vi "Feasa Read Blinking, Colour, Intensity with Options.vi"(0 "VISA in":refnum<visa-resource-name>="COM12", 1 "Capture Time (ms)":i32=200 min=1 max=999, 2 "Exposure Factor":i32=1 caption="(00-15)" format="%02.0f", 3 "Wait Time between Capture (ms)":i32 min=0 max=999, 4 "Number of Capture":i32=20 min=0 max=9999, 5 "error in (no error)":errorcluster, 6 "Fiber Num":T1(ring)=enum."1", 7 "Lower Limit":dbl=2000.0 format="%#_13g", 8 "Maximum/Average/Minimum":enum16{"Maximum", "Average", "Minimum"}(ring), 9 "Upper Limit":dbl=5000.0 format="%#_13g") -> (10 "RED?":bool, 11 "Intensity":i32, 12 "GREEN?":bool, 14 "YELLOW?":bool, 15 "Blinking?":bool, 17 "ON?":bool, 18 "OFF?":bool, 19 "error out":errorcluster)   [LabVIEW 2025]
doc: "This VI is to for LED testwith using FEASA sequence mode.\n\nInput:\n- VISA in:\n Comm port in.\n\n- Fiber Num:\n Select Fiber Number to test. Fiber 1 to 10 channel. (can use for LED Analyser in 3F and 10F) \n\n- Capture Time (ms):\n Set capture time in milliseconds. \n (Note : This depends on the brightness of the LED. If the LED is dim then 1mS will cause the Analyser to be under-range. This could be determined by experiment.)\n\n- Wait Time between capture (ms):\n Set Wait time between Capture in milliseconds. \n\n- Number of Capture:\n Set a number of capture.\n\n- Maximum/Average/Minimum:\n Select intensity data and Wavelength to show in maximum value, average or minimum value. Default is maximum value.\n\n- Error in:\n Error message in.\n\nOutput:\n- Wavelength:\n Wavelength measurement (nm).\n\n- Intensity:\n Intensity measurement in count. This is relative intensity.\n\n- Status:\n Sending command process status.\n True : Passed\n False : Failed\n\n- LED Color:\n 1) RED?\n True: Yes.\n False: No.\n 2) GREEN?\n True: Yes.\n False: No.\n 3) BLUE?\n True: Yes.\n False: No.\n\n- LED Status:\n 1) Blinking?\n True: Yes.\n False: No.\n 2) ON?\n True: Yes.\n False: No.\n 3) OFF?\n True: Yes.\n False: No.\n\n- Error out:\n Error message out."
panel:
  out "Wavelength":i32
  out "Intensity (Min)":i32
  out "Wavelength (Min)":i32
  out "Wavelength (Ave)":dbl
  out "Wavelength (Max)":i32
  out "Intensity (Ave)":dbl
  out "Intensity (Max)":i32
  out "Status":bool
  out "Wavelength & Intensity":string
  # "LED Color"
  # "LED Status"
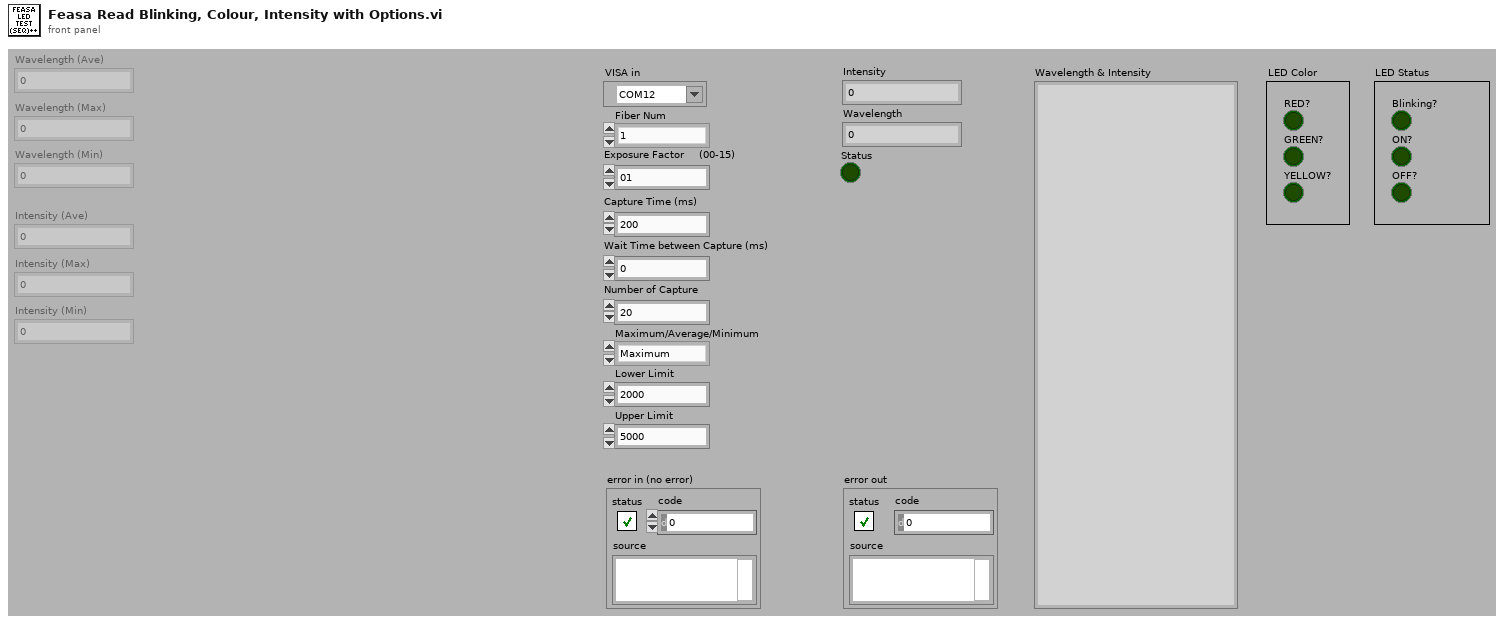
[diagram p1: front panel]
types:
  T1 = enum16{"All", "1", "2", "3", "4", "5", "6", "7", "8", "9", "10"}
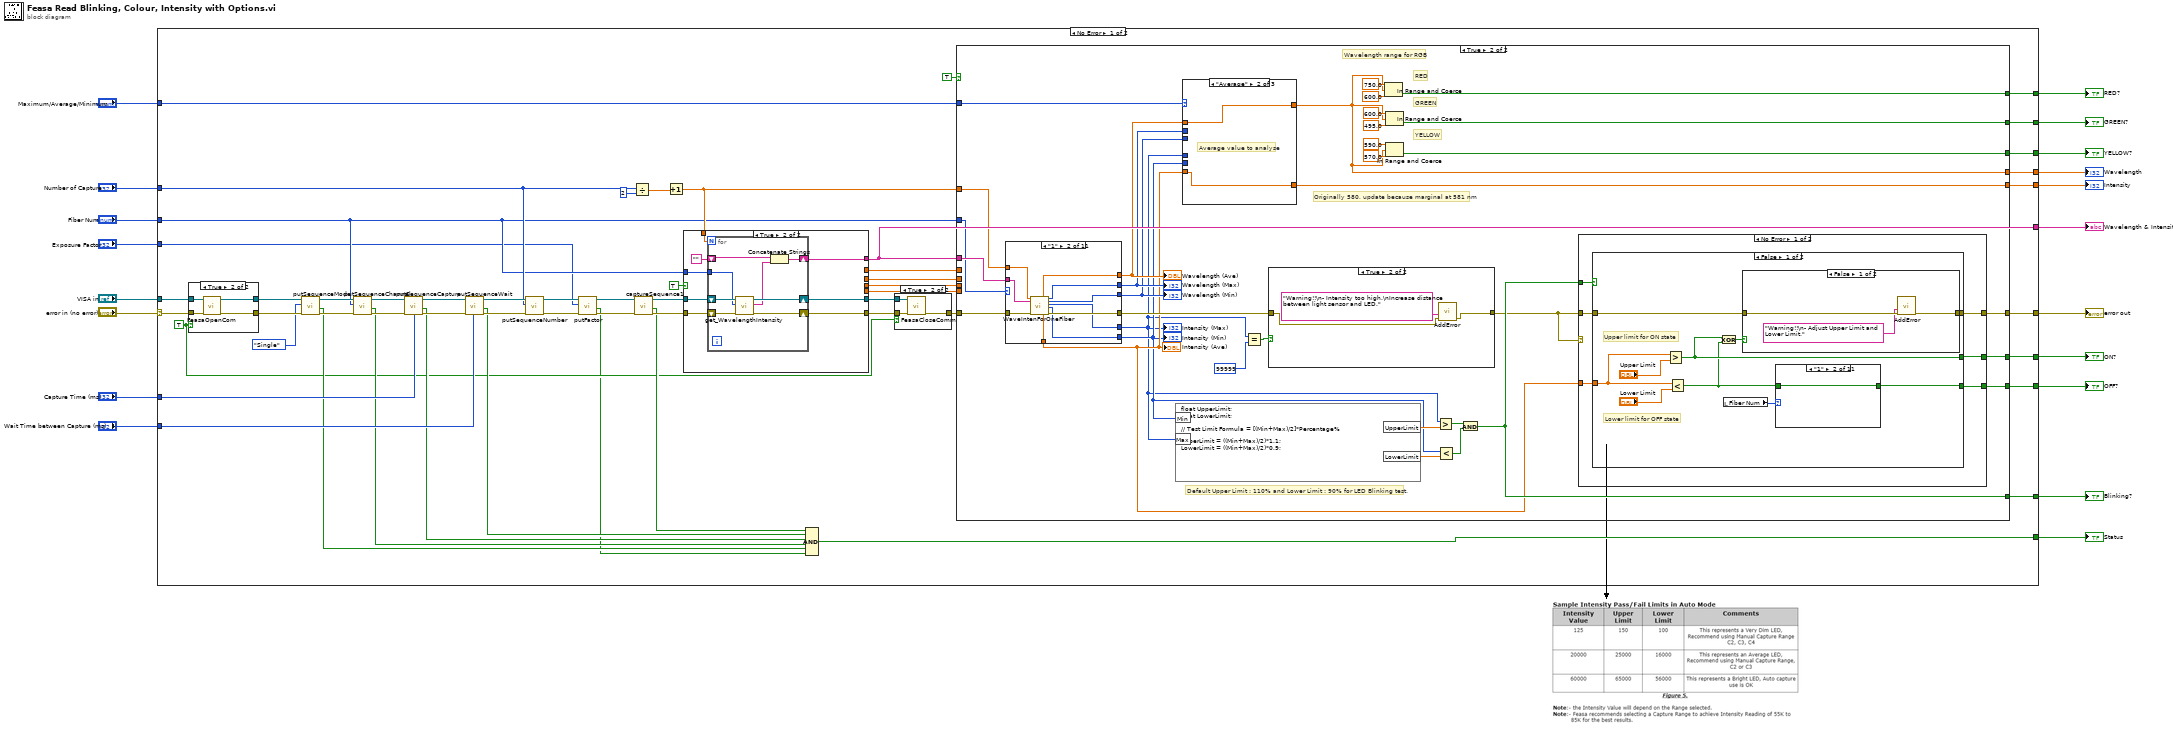
[diagram p0: block diagram]
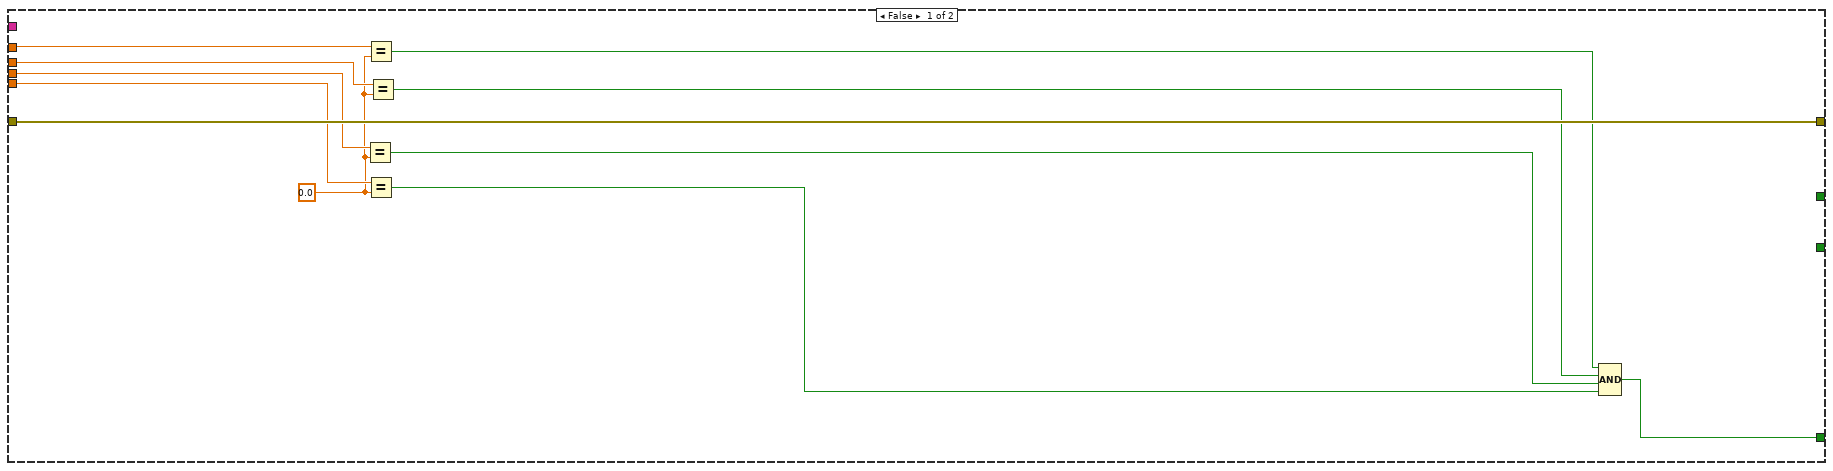
[diagram p4: hidden frame]
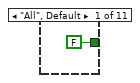
[diagram p5: hidden frame]
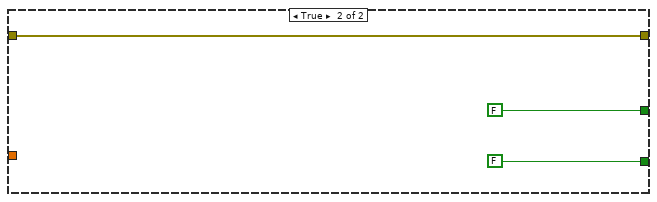
[diagram p16: hidden frame]
diagram:
  n1 = case shown="No Error" "error in (no error)" {
    selector: "error in (no error)" -> [w73 w301]
    tunnel: "VISA in" -> [w74 _]
    tunnel: [w41 w301] -> w17
    tunnel: "Fiber Num" -> [w36 _]
    tunnel: "Capture Time (ms)" -> [w70 _]
    tunnel: "Wait Time between Capture (ms)" -> [w67 _]
    tunnel: "Number of Capture" -> [w60 _]
    tunnel: [w52 _] -> w12
    tunnel: [w54 _] -> w11
    tunnel: "Maximum/Average/Minimum" -> [w50 _]
    tunnel: [w49 _] -> w9
    tunnel: [w48 _] -> w8
    tunnel: [w47 _] -> w7
    tunnel: [w46 _] -> w6
    tunnel: [w45 _] -> w5
    tunnel: [w44 _] -> w4
    tunnel: [w43 _] -> w3
    tunnel: [w42 _] -> w2
    tunnel: "Exposure Factor" -> [w21 _]
    frame No Error {
      w26 = TRUE
      n2 = case shown="True" w26 {
        tunnel: w74 -> [w79 w84]
        tunnel: w73 -> [w80 w83]
        tunnel: [w79 w82] -> w72
        tunnel: [w80 w81] -> w71
        frame False {
        }
        frame True {
          n3 = call "FeasaOpenCom.vi"("error in (no error)"=w83, "VISA resource name"=w84) -> ("error out"=w81:errorcluster, "VISA out"=w82:refnum<visa-resource-name>)  [unwired: 8 in]
        }
      }
      n4 = call "putSequenceMode.vi"("error in"=w71, "Sequence Mode"=enum16{"All", "Single"}."Single", "VISA in"=w72) -> ("error out"=w39:errorcluster, "Status"=w34:bool, "VISA out"=w37:refnum<visa-resource-name>)  [unwired: 6 in]
      n5 = call "putSequenceChannel.vi"("error in"=w39, "Fiber Num"=w36, "VISA in"=w37) -> ("error out"=w38:errorcluster, "Status"=w33:bool, "VISA out"=w35:refnum<visa-resource-name>)  [unwired: 6 in]
      n6 = call "putSequenceCapture.vi"("error in"=w38, "Millisecond (ms)"=w70, "VISA in"=w35) -> ("error out"=w68:errorcluster, "Status"=w55:bool, "VISA out"=w69:refnum<visa-resource-name>)  [unwired: 6 in]
      n7 = call "putSequenceWait.vi"("error in"=w68, "Millisecond (ms)"=w67, "VISA in"=w69) -> ("error out"=w65:errorcluster, "Status"=w56:bool, "VISA out"=w66:refnum<visa-resource-name>)  [unwired: 6 in]
      n8 = call "putSequenceNumber.vi"("error in"=w65, "Number to Capture"=w60, "VISA in"=w66) -> ("error out"=w22:errorcluster, "VISA out"=w25:refnum<visa-resource-name>)  [unwired: 6 in, 1 out]
      n9 = call "putFactor.vi"("error in"=w22, "Exposure Factor"=w21, "VISA in"=w25) -> ("error out"=w23:errorcluster, "Status"=w20:bool, "VISA out"=w24:refnum<visa-resource-name>)  [unwired: 6 in]
      n10 = Divide(x=w60, y=2) -> (x/y=w58:dbl)
      n11 = call "captureSequence1.vi"("error in"=w23, "VISA in"=w24) -> ("error out"=w62:errorcluster, "Status"=w57:bool, "VISA out"=w64:refnum<visa-resource-name>)  [unwired: 7 in]
      n12 = Increment(x=w58) -> (x+1=w51:dbl)
      n13 = case shown="True" TRUE {
        tunnel: w64 -> [w282 w292]
        tunnel: [w280 w291] -> w63
        tunnel: w62 -> [w283 w290]
        tunnel: [w284 w289] -> w61
        tunnel: [_ w287] -> w52
        tunnel: w51 -> [_ w286]
        tunnel: w36 -> [w281 w285]
        tunnel: [w279 _] -> w30
        tunnel: [w278 _] -> w29
        tunnel: [w277 _] -> w28
        tunnel: [w276 _] -> w27
        frame False {
          n14 = call "getflicker.vi"("VISA resource name"=w282, "fiber number"=w281, "error in"=w283) -> ("dup VISA resource name"=w280:refnum<visa-resource-name>, "Flicker %"=w279:dbl, "Flicker index"=w278:dbl, "Flicker Frequencies 1"=w277:dbl, "Flicker Frequencies 2"=w276:dbl, "error out"=w284:errorcluster)  [unwired: 11 in]
        }
        frame True {
          n15 = for {
            N: w286 -> [_]
            shift-right: [w299] -> w291
            shift-left: w292 -> [w300]
            shift-right: [w297] -> w289
            shift-left: w290 -> [w298]
            shift-right: [w294] -> w287
            shift-left: "" -> [w296]
            tunnel: w285 -> [w293]
            n16 = call "get_WavelengthIntensity.vi"("error in"=w298, "Fiber Num"=w293, "VISA in"=w300) -> ("error out"=w297:errorcluster, "WAVELENGTH INTENSITY"=w295:string, "VISA out"=w299:refnum<visa-resource-name>)  [unwired: 6 in]
            n17 = Concatenate Strings(w296, w295) -> (w294:string)
          }
        }
      }
      n18 = Compound Arithmetic op=AND(w57, w56, w55, w33, w34, w20) -> (w54:bool)
      n19 = case shown="True" w26 {
        tunnel: w63 -> [_ w78]
        tunnel: w61 -> [w75 w77]
        tunnel: [w75 w76] -> w53
        frame False {
        }
        frame True {
          n20 = call "FeasaCloseComm.vi"("error in"=w77, "VISA in:"=w78) -> ("error out"=w76:errorcluster)  [unwired: 9 in]
        }
      }
      n21 = case shown="True" TRUE {
        tunnel: w53 -> [w95 w129]
        tunnel: w52 -> [_ w128]
        tunnel: w51 -> [_ w127]
        tunnel: w50 -> [_ w121]
        tunnel: [_ w116] -> w49
        tunnel: [_ w115] -> w48
        tunnel: [_ w114] -> w47
        tunnel: [_ w113] -> w46
        tunnel: [_ w112] -> w45
        tunnel: [w89 w106] -> w44
        tunnel: [_ w104] -> w43
        tunnel: [_ w103] -> w42
        tunnel: [w95 w101] -> w41
        tunnel: w36 -> [_ w96]
        tunnel: w30 -> [w94 _]
        tunnel: w29 -> [w93 _]
        tunnel: w28 -> [w92 _]
        tunnel: w27 -> [w91 _]
        frame False {
          w90 = 0.0 ("y")
          n22 = Equal?(x=w92, y=w90) -> (x = y?=w86:bool)
          n23 = Equal?(x=w94, y=w90) -> (x = y?=w88:bool)
          n24 = Equal?(x=w91, y=w90) -> (x = y?=w85:bool)
          n25 = Equal?(x=w93, y=w90) -> (x = y?=w87:bool)
          n26 = Compound Arithmetic op=AND(w88, w87, w86, w85) -> (w89:bool)
        }
        frame True {
          # "Originally 580, update because marginal at 581 nm"
          # "YELLOW"
          # "GREEN"
          # "RED"
          # "Wavelength range for RGB"
          # "Default Upper Limit : 110% and Lower Limit : 90% for LED Blinking test."
          n27 = case shown="\"1\"" w96 {
            tunnel: w129 -> [w175 w185 w195 w205 w215 w225 w235 w245 w255 w265 w275]
            tunnel: [w175 w184 w194 w204 w214 w224 w234 w244 w254 w264 w274] -> w109
            tunnel: w128 -> [_ w183 w193 w203 w213 w223 w233 w243 w253 w263 w273]
            tunnel: w127 -> [_ w182 w192 w202 w212 w222 w232 w242 w252 w262 w272]
            tunnel: [_ w181 w191 w201 w211 w221 w231 w241 w251 w261 w271] -> w120
            tunnel: [_ w180 w190 w200 w210 w220 w230 w240 w250 w260 w270] -> w119
            tunnel: [_ w179 w189 w199 w209 w219 w229 w239 w249 w259 w269] -> w118
            tunnel: [_ w178 w188 w198 w208 w218 w228 w238 w248 w258 w268] -> w97
            tunnel: [_ w177 w187 w197 w207 w217 w227 w237 w247 w257 w267] -> w98
            tunnel: [_ w176 w186 w196 w206 w216 w226 w236 w246 w256 w266] -> w105
            frame "All", Default {
            }
            frame "1" {
              n28 = call "WaveIntenForOneFiber.vi"("Number of Data"=w182, "String Input"=w183, "error in"=w185) -> ("Wavelength (Ave)"=w181:dbl, "Intensity (Ave)"=w176:dbl, "Wavelength (Max)"=w180:i32, "Wavelength (Min)"=w179:i32, "Intensity (Max)"=w178:i32, "Intensity (Min)"=w177:i32, "error out"=w184:errorcluster)  [unwired: 10 in]
            }
            frame "2" {
              n29 = call "WaveIntenForOneFiber.vi"("Number of Data"=w192, "String Input"=w193, "error in"=w195) -> ("Wavelength (Ave)"=w191:dbl, "Intensity (Ave)"=w186:dbl, "Wavelength (Max)"=w190:i32, "Wavelength (Min)"=w189:i32, "Intensity (Max)"=w188:i32, "Intensity (Min)"=w187:i32, "error out"=w194:errorcluster)  [unwired: 10 in]
            }
            frame "3" {
              n30 = call "WaveIntenForOneFiber.vi"("Number of Data"=w202, "String Input"=w203, "error in"=w205) -> ("Wavelength (Ave)"=w201:dbl, "Intensity (Ave)"=w196:dbl, "Wavelength (Max)"=w200:i32, "Wavelength (Min)"=w199:i32, "Intensity (Max)"=w198:i32, "Intensity (Min)"=w197:i32, "error out"=w204:errorcluster)  [unwired: 10 in]
            }
            frame "4" {
              n31 = call "WaveIntenForOneFiber.vi"("Number of Data"=w212, "String Input"=w213, "error in"=w215) -> ("Wavelength (Ave)"=w211:dbl, "Intensity (Ave)"=w206:dbl, "Wavelength (Max)"=w210:i32, "Wavelength (Min)"=w209:i32, "Intensity (Max)"=w208:i32, "Intensity (Min)"=w207:i32, "error out"=w214:errorcluster)  [unwired: 10 in]
            }
            frame "5" {
              n32 = call "WaveIntenForOneFiber.vi"("Number of Data"=w222, "String Input"=w223, "error in"=w225) -> ("Wavelength (Ave)"=w221:dbl, "Intensity (Ave)"=w216:dbl, "Wavelength (Max)"=w220:i32, "Wavelength (Min)"=w219:i32, "Intensity (Max)"=w218:i32, "Intensity (Min)"=w217:i32, "error out"=w224:errorcluster)  [unwired: 10 in]
            }
            frame "6" {
              n33 = call "WaveIntenForOneFiber.vi"("Number of Data"=w232, "String Input"=w233, "error in"=w235) -> ("Wavelength (Ave)"=w231:dbl, "Intensity (Ave)"=w226:dbl, "Wavelength (Max)"=w230:i32, "Wavelength (Min)"=w229:i32, "Intensity (Max)"=w228:i32, "Intensity (Min)"=w227:i32, "error out"=w234:errorcluster)  [unwired: 10 in]
            }
            frame "7" {
              n34 = call "WaveIntenForOneFiber.vi"("Number of Data"=w242, "String Input"=w243, "error in"=w245) -> ("Wavelength (Ave)"=w241:dbl, "Intensity (Ave)"=w236:dbl, "Wavelength (Max)"=w240:i32, "Wavelength (Min)"=w239:i32, "Intensity (Max)"=w238:i32, "Intensity (Min)"=w237:i32, "error out"=w244:errorcluster)  [unwired: 10 in]
            }
            frame "8" {
              n35 = call "WaveIntenForOneFiber.vi"("Number of Data"=w252, "String Input"=w253, "error in"=w255) -> ("Wavelength (Ave)"=w251:dbl, "Intensity (Ave)"=w246:dbl, "Wavelength (Max)"=w250:i32, "Wavelength (Min)"=w249:i32, "Intensity (Max)"=w248:i32, "Intensity (Min)"=w247:i32, "error out"=w254:errorcluster)  [unwired: 10 in]
            }
            frame "9" {
              n36 = call "WaveIntenForOneFiber.vi"("Number of Data"=w262, "String Input"=w263, "error in"=w265) -> ("Wavelength (Ave)"=w261:dbl, "Intensity (Ave)"=w256:dbl, "Wavelength (Max)"=w260:i32, "Wavelength (Min)"=w259:i32, "Intensity (Max)"=w258:i32, "Intensity (Min)"=w257:i32, "error out"=w264:errorcluster)  [unwired: 10 in]
            }
            frame "10" {
              n37 = call "WaveIntenForOneFiber.vi"("Number of Data"=w272, "String Input"=w273, "error in"=w275) -> ("Wavelength (Ave)"=w271:dbl, "Intensity (Ave)"=w266:dbl, "Wavelength (Max)"=w270:i32, "Wavelength (Min)"=w269:i32, "Intensity (Max)"=w268:i32, "Intensity (Min)"=w267:i32, "error out"=w274:errorcluster)  [unwired: 10 in]
            }
          }
          "Intensity (Max)" <- w97
          "Intensity (Ave)" <- w105
          "Wavelength (Max)" <- w119
          "Wavelength (Ave)" <- w120
          "Wavelength (Min)" <- w118
          "Intensity (Min)" <- w98
          n38 = formula code="float UpperLimit;\nfloat LowerLimit;\n\n// Test Limit Formula = [(Min+Max)/2]*Percentage%\n\nUpperLimit = ((Min+Max)/2)*1.1;  \nLowerLimit = ((Min+Max)/2)*0.9;"("Min"=w98, "Max"=w97) -> ("UpperLimit"=w100:dbl, "LowerLimit"=w99:dbl)
          n39 = case shown="\"Average\"" w121 {
            tunnel: w120 -> [_ w172 _]
            tunnel: w119 -> [w170 _ _]
            tunnel: w118 -> [_ _ w174]
            tunnel: w97 -> [w169 _ _]
            tunnel: w98 -> [_ _ w173]
            tunnel: w105 -> [_ w171 _]
            tunnel: [w170 w172 w174] -> w113
            tunnel: [w169 w171 w173] -> w112
            frame "Maximum", Default {
              # "Maximum value to analyse"
            }
            frame "Average" {
              # "Average value to analyse"
            }
            frame "Minimum" {
              # "Minimum value to analyse"
            }
          }
          n40 = Equal?(x=w97, y=99999) -> (x = y?=w111:bool)
          n41 = case shown="True" w111 {
            tunnel: w109 -> [w165 w167]
            tunnel: [w165 w168] -> w102
            frame False {
            }
            frame True {
              n42 = call "AddError.vi"("error in"=w167, "Error Message"="Warning!!\n- Intensity too high.\nIncrease distance between light sensor and LED." ("message")) -> ("error out"=w168:errorcluster)  [unwired: 9 in]
            }
          }
          n43 = In Range and Coerce(upper limit=750.0, x=w113, lower limit=600.0) -> (In Range?=w116:bool)  [unwired: 1 out]
          n44 = In Range and Coerce(upper limit=600.0, x=w113, lower limit=495.0) -> (In Range?=w115:bool)  [unwired: 1 out]
          n45 = In Range and Coerce(upper limit=590.0, x=w113, lower limit=570.0) -> (In Range?=w114:bool)  [unwired: 1 out]
          n46 = Greater?(x=w97, y=w100) -> (0:w108:bool)
          n47 = Less?(x=w98, y=w99) -> (x < y?=w107:bool)
          n48 = And(x=w108, y=w107) -> (x .and. y?=w106:bool)
          n49 = case shown="No Error" w102 {
            tunnel: w106 -> [w135 _]
            tunnel: w105 -> [w134 _]
            tunnel: [w133 _] -> w104
            tunnel: [w132 _] -> w103
            tunnel: [w130 w164] -> w101
            tunnel: w102 -> [w131 w164]
            frame No Error {
              n50 = case shown="False" w135 {
                tunnel: w134 -> [w140 _]
                tunnel: [w143 FALSE] -> w133
                tunnel: [w137 FALSE] -> w132
                tunnel: [w142 w161] -> w130
                tunnel: w131 -> [w136 w161]
                frame False {
                  # "Lower limit for OFF state"
                  # "Upper limit for ON state"
                  n51 = Greater?(x=w140, y="Upper Limit") -> (0:w143:bool)
                  n52 = Less?(x=w140, y="Lower Limit") -> (x < y?=w138:bool)
                  n53 = Exclusive Or(1:w138, 2:w143) -> (0:w141:bool)
                  n54 = local read "Fiber Num"() -> (w139:T1)
                  n55 = case shown="False" w141 {
                    tunnel: [w159 w160] -> w142
                    tunnel: w136 -> [w158 w160]
                    frame False {
                      n56 = call "AddError.vi"("error in"=w158, "Error Message"="Warning!!\n- Adjust Upper Limit and Lower Limit." ("message")) -> ("error out"=w159:errorcluster)  [unwired: 9 in]
                    }
                    frame True {
                    }
                  }
                  n57 = case shown="\"1\"" w139 {
                    tunnel: w138 -> [_ w147 w148 w149 w150 w151 w152 w153 w154 w155 w156]
                    tunnel: [FALSE w147 w148 w149 w150 w151 w152 w153 w154 w155 w156] -> w137
                    frame "All", Default {
                    }
                    frame "1" {
                    }
                    frame "2" {
                    }
                    frame "3" {
                    }
                    frame "4" {
                    }
                    frame "5" {
                    }
                    frame "6" {
                    }
                    frame "7" {
                    }
                    frame "8" {
                    }
                    frame "9" {
                    }
                    frame "10" {
                    }
                  }
                }
                frame True {
                }
              }
            }
            frame Error {
            }
          }
        }
      }
    }
    frame Error {
    }
  }
  "error out" <- w17
  "Wavelength & Intensity" <- w12
  "Status" <- w11
  "RED?" <- w9
  "GREEN?" <- w8
  "YELLOW?" <- w7
  "Wavelength" <- w6
  "Intensity" <- w5
  "Blinking?" <- w4
  "ON?" <- w3
  "OFF?" <- w2
